vi "Build Do Interface.vi"(6 "Wiring Spec":T2, 8 "error in (no error)":errorcluster, 9 "AF Library FQN":string, 10 "References":T1, 11 "Do VI":refnum<vi>) -> (0 "error out":errorcluster)   [LabVIEW 2023, in "Message Maker.lvclass"]
doc: "Builds Do.vi for the new message\n\nAuthor: Derek Trepanier\nCopyright: MGI 2015"
uses:
  Message Maker.lvclass
  Wiring Spec.ctl
  Connector Pane Position.ctl
  Scripting Refs.ctl
  <vilib>/Utility/traverseref.llb/TRef TravTarget.ctl
  <vilib>/Utility/miscctls.llb/LVPointTypeDef.ctl
  a1bd7a8b-8878-48b3-8598-ae92486997e2.vi
  <vilib>/Utility/traverseref.llb/VI Scripting - Traverse.lvlib
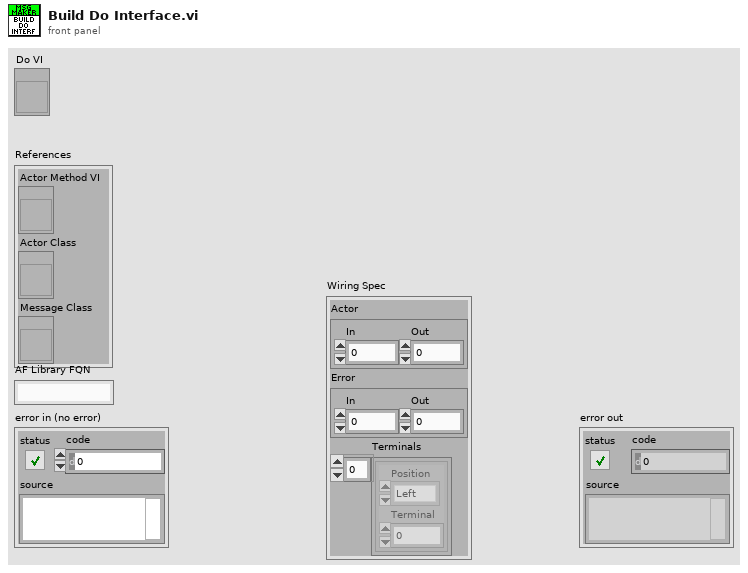
[diagram p1: front panel]
types:
  T1 = typedef "Message Maker.lvclass/Scripting Refs.ctl" = cluster{"Actor Method VI":refnum<vi>, "Actor Class":refnum<vi>, "Message Class":refnum<vi>}
  T2 = typedef "Message Maker.lvclass/Wiring Spec.ctl" = cluster{"Actor":cluster{"In":i32, "Out":i32}, "Error":cluster{"In":i32, "Out":i32}, "Terminals":cluster{"Position":T3, "Terminal":i32}[]}
  T3 = typedef "Message Maker.lvclass/Connector Pane Position.ctl" = enum16{"Left", "Top", "Bottom", "Right"}
  T4 = enum16{"Replace Class Controls/Constants", "Wire Special Inputs", "Wire Outputs", "Wire Method Inputs", "Connect Unbundler Input", "Change for PPL"}
  T5 = typedef "TRef TravTarget.ctl" = enum16{"FP", "BD", "Other"}
  T6 = typedef "LVPointTypeDef.ctl" = cluster{"Horizontal":i16, "Vertical":i16}
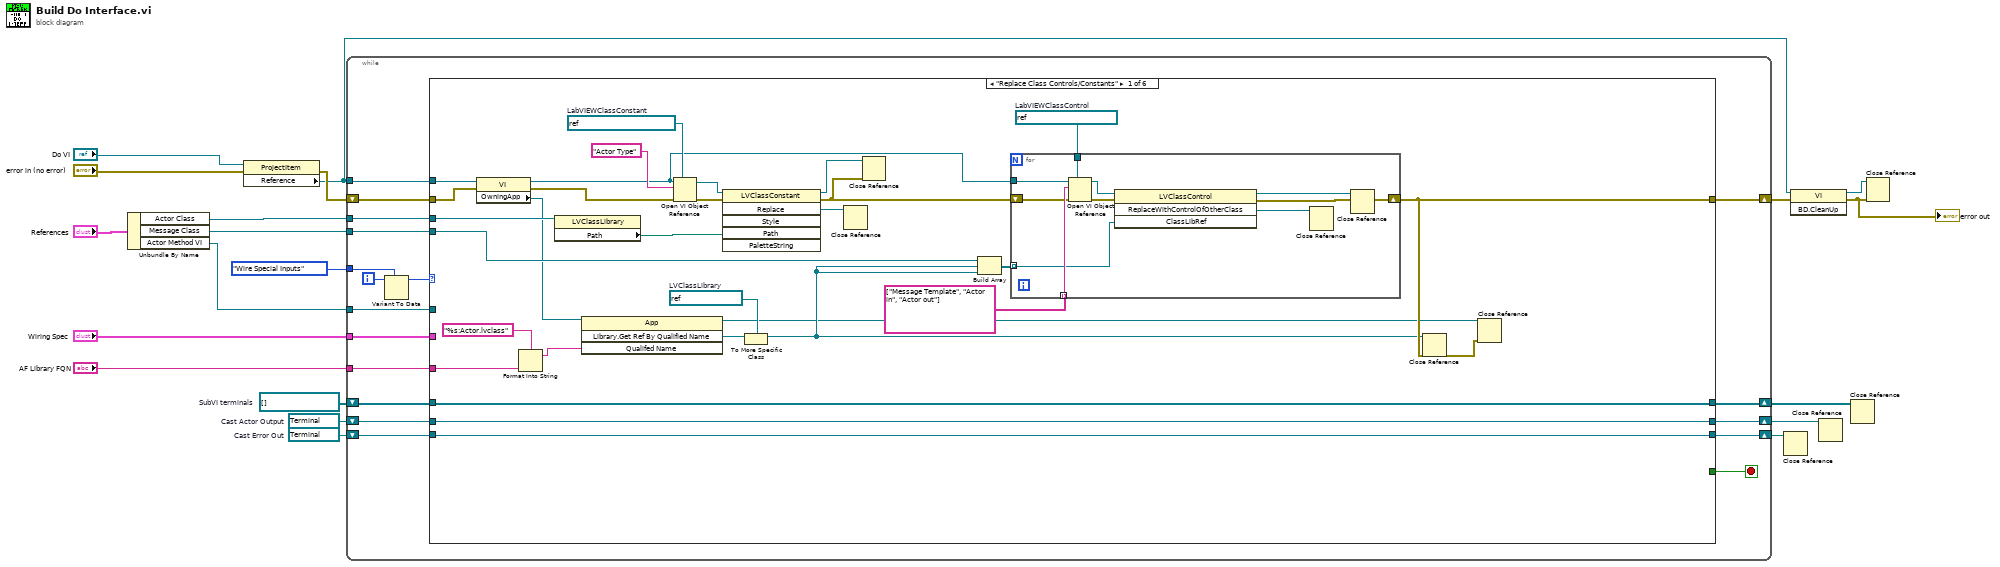
[diagram p0: block diagram]
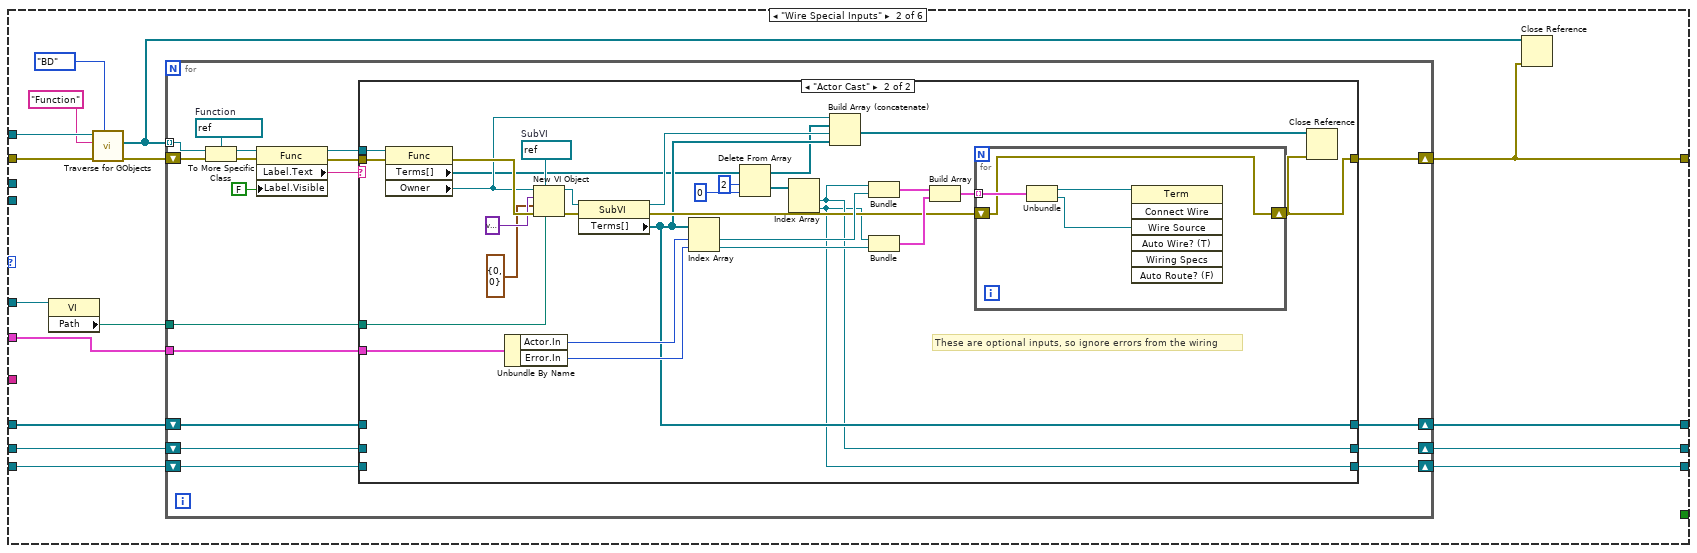
[diagram p2: hidden frame]
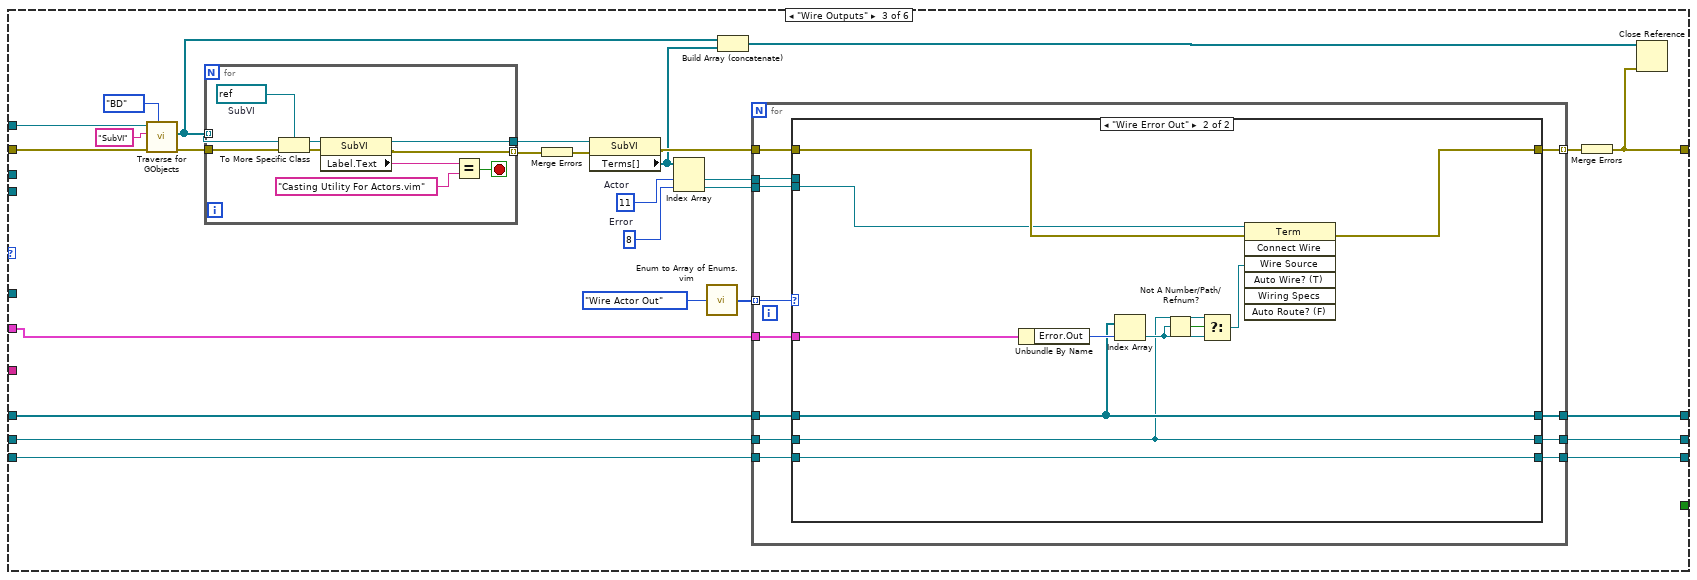
[diagram p4: hidden frame]
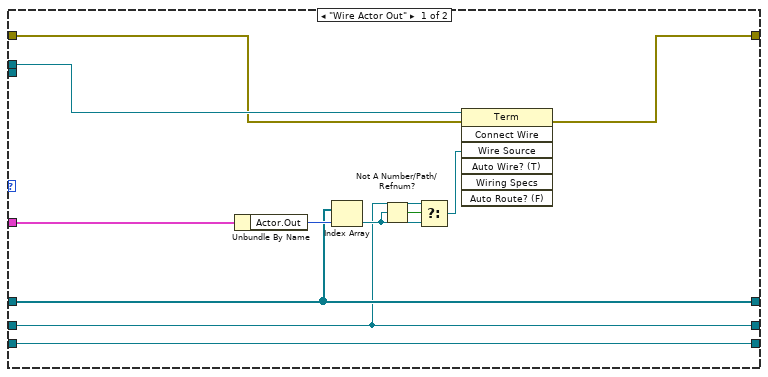
[diagram p5: hidden frame]
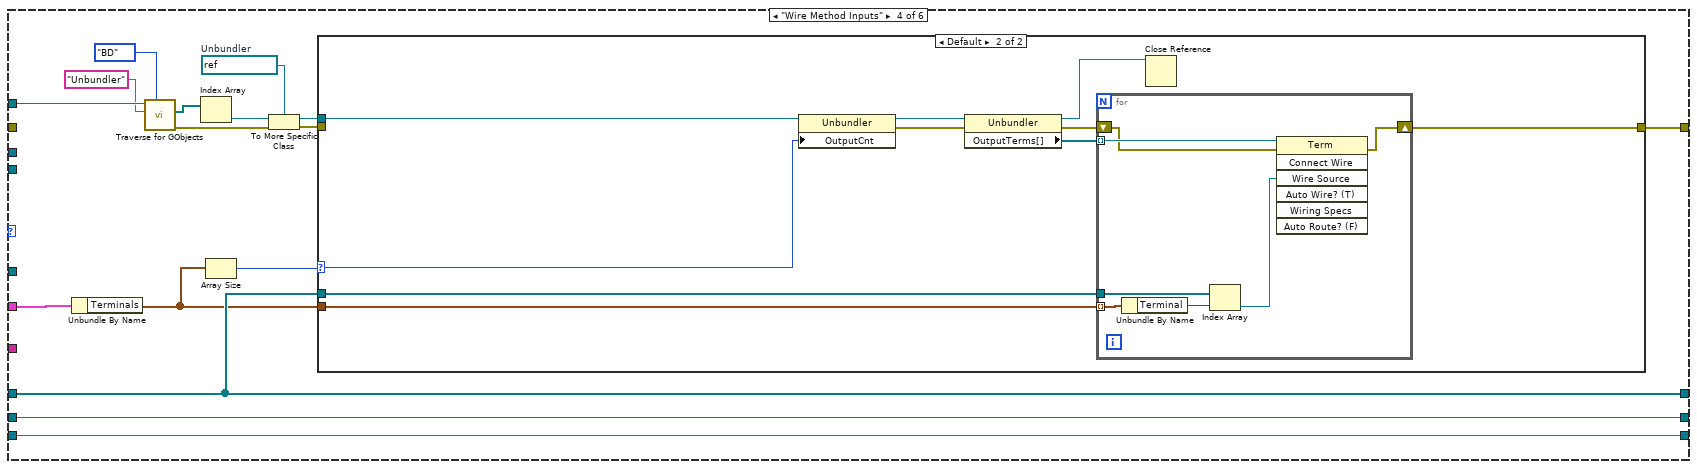
[diagram p6: hidden frame]
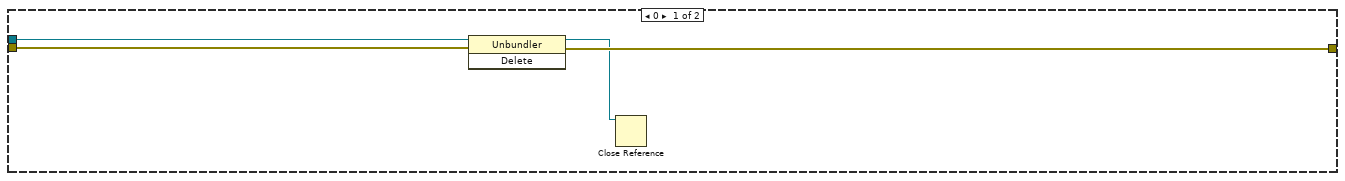
[diagram p7: hidden frame]
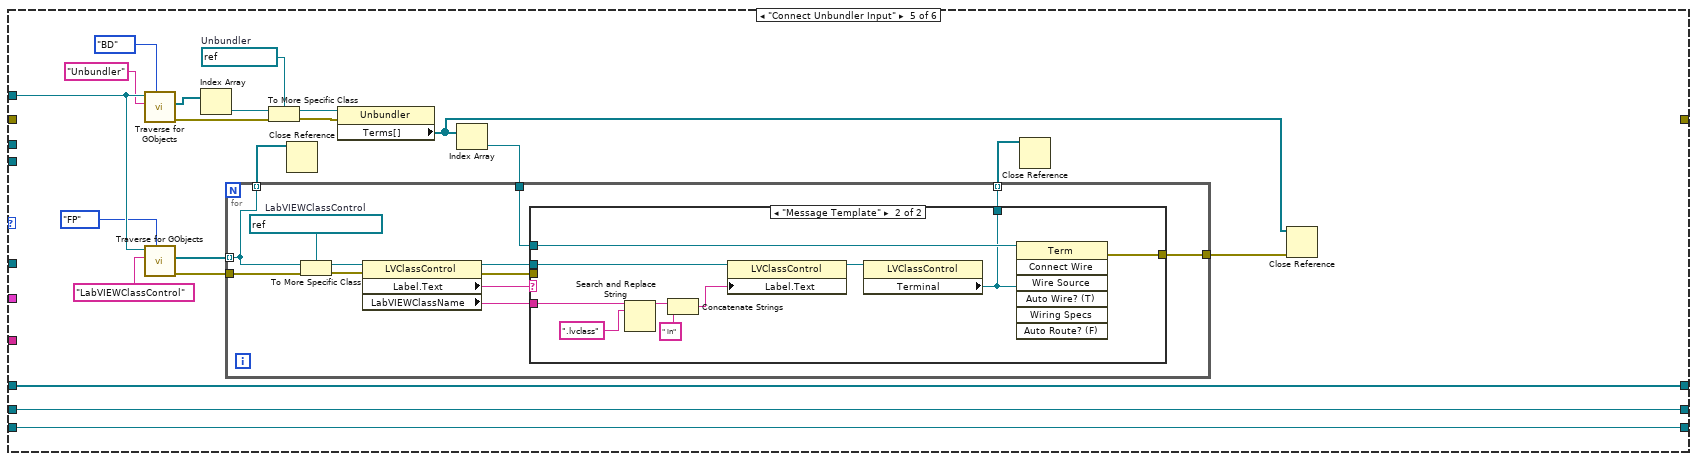
[diagram p8: hidden frame]
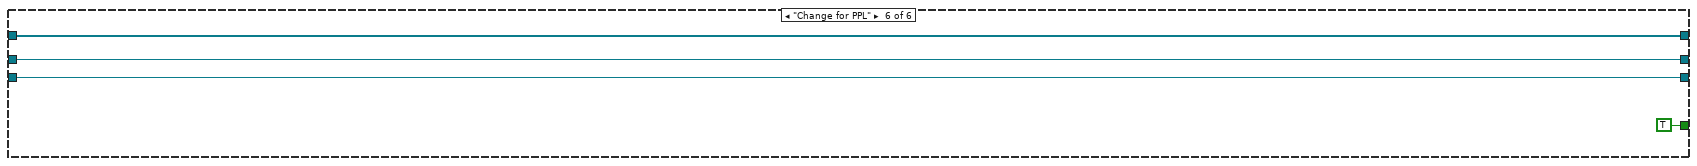
[diagram p10: hidden frame]
diagram:
  w8 = refnum<vi> refnum  # Cast Error Out
  w9 = refnum<vi> refnum  # Cast Actor Output
  w13 = refnum<vi>[] []  # SubVI terminals
  n1 = Unbundle By Name("References") -> ("Actor Class"=w4:refnum<vi>, "Message Class"=w2:refnum<vi>, "Actor Method VI"=w3:refnum<vi>)
  n2 = property class="ProjectItem"(reference="Do VI", error in="error in (no error)") -> (error out=w19:errorcluster, "Reference"=w11:refnum<vi>)  [unwired: 1 out]
  n3 = while {
    tunnel: w11 -> [w38]
    tunnel: "Wiring Spec" -> [w36]
    shift-right: [w35] -> w16
    shift-left: w19 -> [w37]
    tunnel: T4."Wire Special Inputs" -> [w33]
    tunnel: w4 -> [w31]
    tunnel: w3 -> [w30]
    shift-right: [w28] -> w12
    shift-left: w13 -> [w27]
    shift-right: [w26] -> w7
    shift-left: w9 -> [w24]
    shift-right: [w25] -> w6
    shift-left: w8 -> [w23]
    tunnel: w2 -> [w22]
    tunnel: "AF Library FQN" -> [w21]
    i -> [w34]
    stop <- w29 stop-if-true
    n4 = Variant To Data(type=w33, Variant=w34) -> (data=w32:T4)  [unwired: 1 in, 1 out]
    n5 = case shown="\"Replace Class Controls/Constants\"" w32 {
      tunnel: w38 -> [w60 w94 w151 w237 w279 _]
      tunnel: w37 -> [w57 w92 w167 _ _ _]
      tunnel: w36 -> [_ w90 w156 w230 _ _]
      tunnel: [w42 w86 w152 w226 _ _] -> w35
      tunnel: w31 -> [w65 _ _ _ _ _]
      tunnel: w30 -> [_ w87 _ _ _ _]
      tunnel: [_ _ _ _ _ TRUE] -> w29
      tunnel: [w63 w84 w163 w225 w278 w304] -> w28
      tunnel: w27 -> [w63 w83 w166 w225 w278 w304]
      tunnel: [w62 w82 w162 w224 w277 w303] -> w26
      tunnel: [w61 w81 w161 w223 w276 w302] -> w25
      tunnel: w24 -> [w62 w80 w165 w224 w277 w303]
      tunnel: w23 -> [w61 w79 w164 w223 w276 w302]
      tunnel: w22 -> [w59 _ _ _ _ _]
      tunnel: w21 -> [w45 _ _ _ _ _]
      frame "Replace Class Controls/Constants" {
        w46 = refnum<vi> refnum  # LVClassLibrary
        w53 = refnum<vi> refnum  # LabVIEWClassConstant
        w52 = refnum<vi> refnum  # LabVIEWClassControl
        n6 = property class="VI"(reference=w60, error in=w57) -> (reference out=w50:refnum<vi>, error out=w56:errorcluster, "OwningApp"=w48:refnum<vi>)
        n7 = Format Into String(format string="%s:Actor.lvclass", w45) -> (resulting string=w43:string)  [unwired: 2 in, 1 out]
        n8 = property class="LVClassLibrary"(reference=w65) -> ("Path"=w67:path)  [unwired: 1 in, 2 out]
        n9 = invoke class="App" method="Library.Get Ref By Qualified Name"(reference=w48, "Qualifed Name"=w43) -> (reference out=w40:refnum<vi>, "Library.Get Ref By Qualified Name"=w47:refnum<vi>)  [unwired: 2 in, 2 out]
        n10 = Open VI Object Reference(7:w53, 8:w56, 10:"Actor Type" ("Class Name"), 11:w50) -> (0:w68:errorcluster, 3:w55:refnum<vi>)
        n11 = invoke class="LVClassConstant" method="Replace"(reference=w55, error in=w68, "Path"=w67) -> (reference out=w54:refnum<vi>, error out=w49:errorcluster, "Replace"=w64:refnum<vi>)  [unwired: 3 in, 3 out]
        n12 = To More Specific Class(target class=w46, reference=w47) -> (specific class reference=w41:refnum<vi>)  [unwired: 1 in, 1 out]
        n13 = Close Reference(reference=w64) -> ()  [unwired: 1 in, 1 out]
        n14 = Close Reference(reference=w54, error in (no error)=w49) -> ()  [unwired: 1 out]
        n15 = Build Array(w59, w41, w41) -> (w58:refnum<vi>[])
        n16 = for {
          tunnel: w58 -> [w69] mode=indexing
          tunnel: w52 -> [w76]
          tunnel: string[] ["Message Template", "Actor in", "Actor out"] -> [w74] mode=indexing
          tunnel: w50 -> [w73]
          shift-right: [w71] -> w42
          shift-left: w49 -> [w70]
          n17 = Open VI Object Reference(7:w76, 8:w70, 10:w74, 11:w73) -> (0:w75:errorcluster, 3:w77:refnum<vi>)
          n18 = invoke class="LVClassControl" method="ReplaceWithControlOfOtherClass"(reference=w77, error in=w75, "ClassLibRef"=w69) -> (reference out=w72:refnum<vi>, error out=w71:errorcluster, "ReplaceWithControlOfOtherClass"=w78:refnum<vi>)  [unwired: 1 in, 1 out]
          n19 = Close Reference(reference=w78) -> ()  [unwired: 1 in, 1 out]
          n20 = Close Reference(reference=w72) -> ()  [unwired: 1 in, 1 out]
        }
        n21 = Close Reference(reference=w41, error in (no error)=w42) -> (error out=w39:errorcluster)
        n22 = Close Reference(reference=w40, error in (no error)=w39) -> ()  [unwired: 1 out]
      }
      frame "Wire Special Inputs" {
        n23 = property class="VI"(reference=w87) -> ("Path"=w88:path)  [unwired: 1 in, 2 out]
        n24 = call <vilib>:"Traverse for GObjects.vi"("Traverse Target"=TRef_TravTarget."BD", "error in (no error)"=w92, "Class Name"="Function", "VI Refnum"=w94) -> ("error out"=w91:errorcluster, "References"=w85:refnum<vi>[])  [unwired: 4 in, 2 out]
        n25 = for {
          tunnel: w85 -> [w110] mode=indexing
          tunnel: w88 -> [w105]
          tunnel: w90 -> [w103]
          shift-right: [w102] -> w86
          shift-left: w91 -> [w111]
          shift-right: [w100] -> w84
          shift-left: w83 -> [w99]
          shift-right: [w98] -> w82
          shift-left: w80 -> [w96]
          shift-right: [w97] -> w81
          shift-left: w79 -> [w95]
          w112 = refnum<vi> refnum  # Function
          n26 = To More Specific Class(target class=w112, reference=w110, error in=w111) -> (specific class reference=w109:refnum<vi>, error out=w108:errorcluster)
          n27 = property class="Func"(reference=w109, error in=w108, "Label.Visible"=FALSE) -> (reference out=w106:refnum<vi>, error out=w104:errorcluster, "Label.Text"=w107:string)
          n28 = case shown="\"Actor Cast\"" w107 {
            tunnel: w106 -> [_ w146]
            tunnel: w105 -> [_ w145]
            tunnel: w104 -> [w116 w143]
            tunnel: w103 -> [_ w138]
            tunnel: [w116 w127] -> w102
            tunnel: [w115 w124] -> w100
            tunnel: w99 -> [w115 _]
            tunnel: [w114 w118] -> w98
            tunnel: [w113 w117] -> w97
            tunnel: w96 -> [w114 _]
            tunnel: w95 -> [w113 _]
            frame Default {
            }
            frame "Actor Cast" {
              w144 = refnum<vi> refnum  # SubVI
              # "These are optional inputs, so ignore errors from the wiring"
              n29 = property class="Func"(reference=w146, error in=w143) -> (error out=w142:errorcluster, "Terms[]"=w123:refnum<vi>[], "Owner"=w125:refnum<vi>)  [unwired: 1 out]
              n30 = Unbundle By Name(w138) -> ("Actor.In"=w137:i32, "Error.In"=w136:i32)
              n31 = New VI Object(vi object class=w144, owner refnum=w125, style=variant, position/next to=T6 {"Horizontal"=0, "Vertical"=0} ("location"), 6:w145, 8:w142) -> (object refnum=w140:refnum<vi>, 0:w139:errorcluster)  [unwired: 2 in]
              n32 = property class="SubVI"(reference=w140, error in=w139) -> (reference out=w126:refnum<vi>, error out=w130:errorcluster, "Terms[]"=w124:refnum<vi>[])
              n33 = Index Array(array=w124, index #1=w137, index #2=w136) -> (element #1=w135:refnum<vi>, element #2=w134:refnum<vi>)
              n34 = Delete From Array(array=w123, length=2, index=0) -> (deleted portion=w119:refnum<vi>[], array with subset deleted=w121:refnum<vi>[])
              n35 = Index Array(array=w119) -> (element #1=w118:refnum<vi>, element #2=w117:refnum<vi>)  [unwired: 2 in]
              n36 = Build Array (concatenate)(w125, w121, w126, w124) -> (w128:refnum<vi>[])
              n37 = Bundle(w118, w135) -> (w133:cluster{refnum<vi>, refnum<vi>})  [unwired: 1 in]
              n38 = Bundle(w117, w134) -> (w132:cluster{refnum<vi>, refnum<vi>})  [unwired: 1 in]
              n39 = Build Array(w133, w132) -> (w131:cluster{refnum<vi>, refnum<vi>}[])
              n40 = for {
                tunnel: w131 -> [w150] mode=indexing
                shift-right: [w148] -> w127
                shift-left: w130 -> [w148]
                n41 = Unbundle(w150) -> (w149:refnum<vi>, w147:refnum<vi>)
                n42 = invoke class="Term" method="Connect Wire"(reference=w149, "Wire Source"=w147) -> ()  [unwired: 5 in, 7 out]
              }
              n43 = Close Reference(reference=w128, error in (no error)=w127) -> ()  [unwired: 1 out]
            }
          }
        }
        n44 = Close Reference(reference=w85, error in (no error)=w86) -> ()  [unwired: 1 out]
      }
      frame "Wire Outputs" {
        w169 = 8  # Error
        w170 = 11  # Actor
        n45 = call <vilib>:"Traverse for GObjects.vi"("Traverse Target"=TRef_TravTarget."BD", "error in (no error)"=w167, "Class Name"="SubVI", "VI Refnum"=w151) -> ("error out"=w173:errorcluster, "References"=w155:refnum<vi>[])  [unwired: 4 in, 2 out]
        n46 = for {
          tunnel: w173 -> [w219]
          tunnel: w155 -> [w221] mode=indexing
          tunnel: [w215] -> w174
          tunnel: [w212] -> w160 mode=indexing
          stop <- w214 stop-if-true
          w220 = refnum<vi> refnum  # SubVI
          n47 = To More Specific Class(target class=w220, reference=w221, error in=w219) -> (specific class reference=w218:refnum<vi>, error out=w213:errorcluster)
          n48 = property class="SubVI"(reference=w218, error in=w213) -> (reference out=w215:refnum<vi>, error out=w212:errorcluster, "Label.Text"=w217:string)
          n49 = Equal?(x=w217, y="Casting Utility For Actors.vim") -> (x = y?=w214:bool)
        }
        n50 = Merge Errors(w160) -> (w159:errorcluster)
        n51 = property class="SubVI"(reference=w174, error in=w159) -> (error out=w158:errorcluster, "Terms[]"=w154:refnum<vi>[])  [unwired: 1 out]
        n52 = Index Array(array=w154, index #1=w170, index #2=w169) -> (element #1=w175:refnum<vi>, element #2=w176:refnum<vi>)
        n53 = call "Enum to Array of Enums.vim"("enum"=enum16{"Wire Actor Out", "Wire Error Out"}."Wire Actor Out") -> ("array of enums"=w177:enum16{"Wire Actor Out", "Wire Error Out"}[])
        n54 = Build Array (concatenate)(w155, w154) -> (w153:refnum<vi>[])
        n55 = for {
          tunnel: w175 -> [w189]
          tunnel: w176 -> [w188]
          tunnel: w177 -> [w178] mode=indexing
          tunnel: w166 -> [w187]
          tunnel: w165 -> [w186]
          tunnel: w164 -> [w185]
          tunnel: [w184] -> w163
          tunnel: [w183] -> w162
          tunnel: [w182] -> w161
          tunnel: w158 -> [w181]
          tunnel: [w180] -> w157 mode=indexing
          tunnel: w156 -> [w179]
          n56 = case shown="\"Wire Error Out\"" w178 {
            tunnel: w189 -> [w193 _]
            tunnel: w188 -> [_ w201]
            tunnel: w187 -> [w196 w207]
            tunnel: w186 -> [w195 w206]
            tunnel: w185 -> [w194 w205]
            tunnel: [w196 w207] -> w184
            tunnel: [w195 w206] -> w183
            tunnel: [w194 w205] -> w182
            tunnel: w181 -> [w192 w204]
            tunnel: [w191 w203] -> w180
            tunnel: w179 -> [w190 w202]
            frame "Wire Actor Out" {
              n57 = Unbundle By Name(w190) -> ("Actor.Out"=w200:i32)
              n58 = Index Array(array=w196, index=w200) -> (element=w198:refnum<vi>)
              n59 = Not A Number/Path/Refnum?(number/path/refnum=w198) -> (NaN/Path/Refnum?=w197:bool)
              n60 = Select(t=w195, s=w197, f=w198) -> (s? t:f=w199:refnum<vi>)
              n61 = invoke class="Term" method="Connect Wire"(reference=w193, error in=w192, "Wire Source"=w199) -> (error out=w191:errorcluster)  [unwired: 4 in, 6 out]
            }
            frame "Wire Error Out" {
              n62 = Unbundle By Name(w202) -> ("Error.Out"=w211:i32)
              n63 = Index Array(array=w207, index=w211) -> (element=w209:refnum<vi>)
              n64 = Not A Number/Path/Refnum?(number/path/refnum=w209) -> (NaN/Path/Refnum?=w208:bool)
              n65 = Select(t=w206, s=w208, f=w209) -> (s? t:f=w210:refnum<vi>)
              n66 = invoke class="Term" method="Connect Wire"(reference=w201, error in=w204, "Wire Source"=w210) -> (error out=w203:errorcluster)  [unwired: 4 in, 6 out]
            }
          }
        }
        n67 = Merge Errors(w157) -> (w152:errorcluster)
        n68 = Close Reference(reference=w153, error in (no error)=w152) -> ()  [unwired: 1 out]
      }
      frame "Wire Method Inputs" {
        w231 = refnum<vi> refnum  # Unbundler
        n69 = Unbundle By Name(w230) -> ("Terminals"=w222:cluster{"Position":T3, "Terminal":i32}[])
        n70 = call <vilib>:"Traverse for GObjects.vi"("Traverse Target"=TRef_TravTarget."BD", "Class Name"="Unbundler", "VI Refnum"=w237) -> ("error out"=w232:errorcluster, "References"=w234:refnum<vi>[])  [unwired: 5 in, 2 out]
        n71 = Index Array(array=w234) -> (element=w233:refnum<vi>)  [unwired: 1 in]
        n72 = Array Size(array=w222) -> (size(s)=w229:i32)
        n73 = To More Specific Class(target class=w231, reference=w233, error in=w232) -> (specific class reference=w228:refnum<vi>, error out=w227:errorcluster)
        n74 = case shown="Default" w229 {
          selector: w229 -> [_ w246]
          tunnel: w228 -> [w241 w244]
          tunnel: w225 -> [_ w249]
          tunnel: w227 -> [w240 _]
          tunnel: [w239 w243] -> w226
          tunnel: w222 -> [_ w251]
          frame 0 {
            n75 = invoke class="Unbundler" method="Delete"(reference=w241, error in=w240) -> (reference out=w238:refnum<vi>, error out=w239:errorcluster)  [unwired: 1 in, 1 out]
            n76 = Close Reference(reference=w238) -> ()  [unwired: 1 in, 1 out]
          }
          frame Default {
            n77 = property class="Unbundler"(reference=w244, "OutputCnt"=w246) -> (reference out=w247:refnum<vi>, error out=w245:errorcluster)  [unwired: 1 in]
            n78 = property class="Unbundler"(reference=w247, error in=w245) -> (reference out=w242:refnum<vi>, error out=w248:errorcluster, "OutputTerms[]"=w250:refnum<vi>[])
            n79 = for {
              tunnel: w251 -> [w253] mode=indexing
              tunnel: w250 -> [w258] mode=indexing
              tunnel: w249 -> [w257]
              shift-right: [w254] -> w243
              shift-left: w248 -> [w255]
              n80 = Unbundle By Name(w253) -> ("Terminal"=w252:i32)
              n81 = Index Array(array=w257, index=w252) -> (element=w256:refnum<vi>)
              n82 = invoke class="Term" method="Connect Wire"(reference=w258, error in=w255, "Wire Source"=w256) -> (error out=w254:errorcluster)  [unwired: 4 in, 6 out]
            }
            n83 = Close Reference(reference=w242) -> ()  [unwired: 1 in, 1 out]
          }
        }
      }
      frame "Connect Unbundler Input" {
        w271 = refnum<vi> refnum  # Unbundler
        n84 = call <vilib>:"Traverse for GObjects.vi"("Traverse Target"=TRef_TravTarget."BD", "Class Name"="Unbundler", "VI Refnum"=w279) -> ("error out"=w272:errorcluster, "References"=w274:refnum<vi>[])  [unwired: 5 in, 2 out]
        n85 = call <vilib>:"Traverse for GObjects.vi"("Traverse Target"=TRef_TravTarget."FP", "Class Name"="LabVIEWClassControl", "VI Refnum"=w279) -> ("error out"=w270:errorcluster, "References"=w263:refnum<vi>[])  [unwired: 5 in, 2 out]
        n86 = Index Array(array=w274) -> (element=w273:refnum<vi>)  [unwired: 1 in]
        n87 = To More Specific Class(target class=w271, reference=w273, error in=w272) -> (specific class reference=w266:refnum<vi>, error out=w265:errorcluster)
        n88 = property class="Unbundler"(reference=w266, error in=w265) -> ("Terms[]"=w260:refnum<vi>[])  [unwired: 2 out]
        n89 = Index Array(array=w260) -> (element=w264:refnum<vi>)  [unwired: 1 in]
        n90 = for {
          tunnel: w270 -> [w291]
          tunnel: [w282] -> w267 mode=indexing
          tunnel: w264 -> [w284]
          tunnel: w263 -> [w282] mode=indexing
          tunnel: [w281] -> w261
          tunnel: [w280] -> w259 mode=indexing
          w290 = refnum<vi> refnum  # LabVIEWClassControl
          n91 = To More Specific Class(target class=w290, reference=w282, error in=w291) -> (specific class reference=w289:refnum<vi>, error out=w288:errorcluster)
          n92 = property class="LVClassControl"(reference=w289, error in=w288) -> (reference out=w286:refnum<vi>, error out=w285:errorcluster, "Label.Text"=w287:string, "LabVIEWClassName"=w283:string)
          n93 = case shown="\"Message Template\"" w287 {
            tunnel: w286 -> [_ w301]
            tunnel: w285 -> [_ _]
            tunnel: w284 -> [_ w300]
            tunnel: w283 -> [_ w296]
            tunnel: [_ w293] -> w281
            tunnel: [_ w292] -> w280
            frame Default {
            }
            frame "Message Template" {
              n94 = Search and Replace String(input string=w296, search string=".lvclass" ("regular expression")) -> (result string=w295:string)  [unwired: 6 in, 3 out]
              n95 = Concatenate Strings(w295, " in" ("string")) -> (w298:string)
              n96 = property class="LVClassControl"(reference=w301, "Label.Text"=w298) -> (reference out=w299:refnum<vi>)  [unwired: 1 in, 1 out]
              n97 = property class="LVClassControl"(reference=w299) -> ("Terminal"=w292:refnum<vi>)  [unwired: 1 in, 2 out]
              n98 = invoke class="Term" method="Connect Wire"(reference=w300, "Wire Source"=w292) -> (error out=w293:errorcluster)  [unwired: 5 in, 6 out]
            }
          }
        }
        n99 = Close Reference(reference=w267) -> ()  [unwired: 1 in, 1 out]
        n100 = Close Reference(reference=w259) -> ()  [unwired: 1 in, 1 out]
        n101 = Close Reference(reference=w260, error in (no error)=w261) -> ()  [unwired: 1 out]
      }
      frame "Change for PPL" {
      }
    }
  }
  n102 = Close Reference(reference=w6) -> ()  [unwired: 1 in, 1 out]
  n103 = invoke class="VI" method="BD.CleanUp"(reference=w11, error in=w16) -> (reference out=w15:refnum<vi>, error out=w10:errorcluster)  [unwired: 1 in, 1 out]
  "error out" <- w10
  n104 = Close Reference(reference=w7) -> ()  [unwired: 1 in, 1 out]
  n105 = Close Reference(reference=w12) -> ()  [unwired: 1 in, 1 out]
  n106 = Close Reference(reference=w15, error in (no error)=w10) -> ()  [unwired: 1 out]
